vi "temp and led.vi"() -> ()   [LabVIEW 2017]
panel:
  out "Low Lighing":bool
  out "LDR Output (V)":dbl
  out "High Temperature":bool
  out "Low Temperature":bool
  out "Thermometer":dbl(slide) scale=0.0..100.0
  out "Temperatue (C)":dbl
  out "Temperature in (mV)":dbl
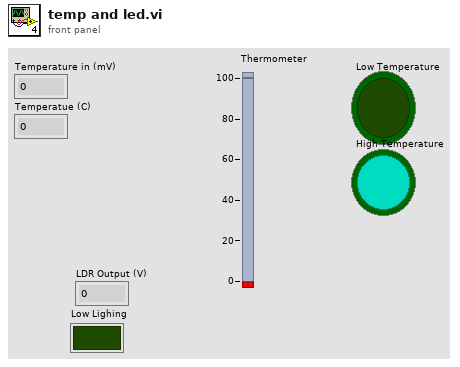
[diagram p1: front panel]
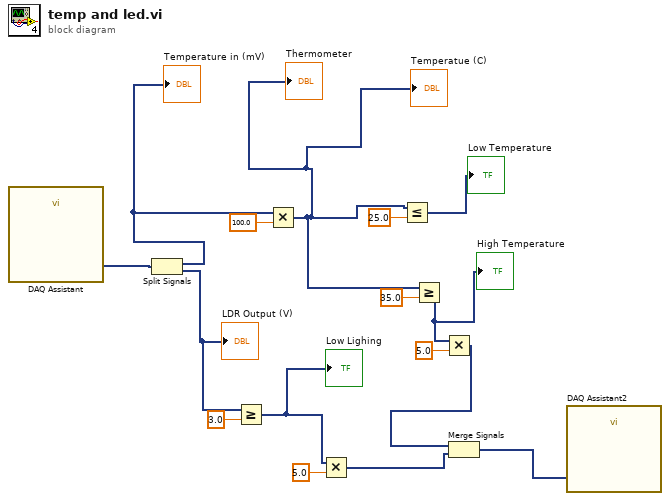
[diagram p0: block diagram]
diagram:
  n1 = call "DAQ Assistant"() -> ("data"=w16:dynamicdata)  [unwired: 16 in, 3 out]
  n2 = Split Signals(w16) -> (w15:dynamicdata, w7:dynamicdata)  [unwired: 2 in]
  "Temperature in (mV)" <- w15
  "LDR Output (V)" <- w7
  n3 = Greater Or Equal?(x=w7, y=3.0) -> (x >= y?=w4:dynamicdata)
  "Low Lighing" <- w4
  n4 = Multiply(x=w15, y=100.0) -> (x*y=w11:dynamicdata)
  "Temperatue (C)" <- w11
  "Thermometer" <- w11
  n5 = Multiply(x=w4, y=5.0) -> (x*y=w2:dynamicdata)
  n6 = Less Or Equal?(x=w11, y=25.0) -> (x <= y?=→"Low Temperature":dynamicdata)
  n7 = Greater Or Equal?(x=w11, y=35.0) -> (x >= y?=w9:dynamicdata)
  "High Temperature" <- w9
  n8 = Multiply(x=w9, y=5.0) -> (x*y=w3:dynamicdata)
  n9 = Merge Signals(w3, w2) -> (w1:dynamicdata)
  n10 = call "DAQ Assistant2"("data"=w1) -> ()  [unwired: 16 in, 3 out]
